vi "GEA2 Register Source Address.vi"(0 "GEA2 Reference In":refnum<k24>, 5 "Old Address":u8, 7 "New Address":u8, 11 "Error In":errorcluster) -> (4 "GEA2 Reference Out":refnum<k24>, 15 "Error Out":errorcluster)   [LabVIEW 2016, in "GEA2_Toolkit.lvlib"]
doc: "This VI unregisters the address you specify and registers a new address on the GEA2 bus."
uses:
  library/GEA2_Toolkit.lvlib
  Q:/Common/LabVIEW GEA2 Toolkit/source/GEA3 DLL Source/GeaCommunication.dll
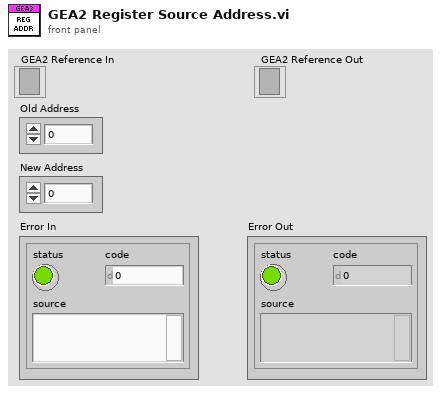
[diagram p1: front panel]
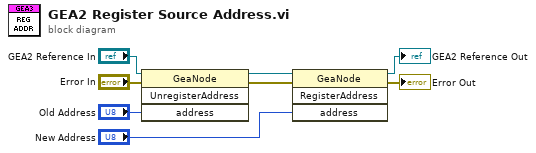
[diagram p0: block diagram]
diagram:
  n1 = invoke class="GeaNode" method="UnregisterAddress"(reference="GEA2 Reference In", error in="Error In", "address"="Old Address") -> (reference out=w5:refnum<k24>, error out=w6:errorcluster)  [unwired: 1 in, 2 out]
  n2 = invoke class="GeaNode" method="RegisterAddress"(reference=w5, error in=w6, "address"="New Address") -> (reference out=→"GEA2 Reference Out":refnum<k24>, error out=→"Error Out":errorcluster)  [unwired: 1 in, 2 out]
